vi "AcqDataQSM.vi"(6 "Temp Notifier":refnum<notifier>, 8 "Pressure Notifier":refnum<notifier>, 9 "Lower Notifier":refnum<notifier>, 10 "Upper Notifier":refnum<notifier>, 11 "Acquisition Control":refnum<queue>) -> ()   [LabVIEW 2013, in "main.lvlib"]
doc: "Læser 4 analoge differentierede datakanaler fra ADC'en og skriver dem til en TDMS-fil. Viser 2 af kanaler i grafer og 2 i søjler."
uses:
  main.lvlib
  Controls/Enum Globals.ctl
  Controls/Enum Variables.ctl
  Controls/Enum User Events.ctl
  <vilib>/DAQmx/read.llb/DAQmx Read (Analog 1D DBL NChan 1Samp).vi
  Globals/DataAcqRecordPathGlobal.vi
  <vilib>/DAQmx/miscellaneous.llb/DAQmx Fill In Error Info.vi
panel:
  in  "input cluster":T1
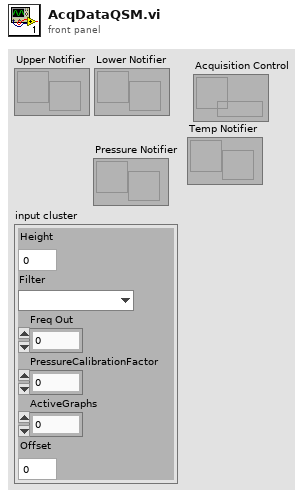
[diagram p1: front panel]
types:
  T1 = cluster{"Height":dbl, "Filter":u16, "Freq Out":i32, "PressureCalibrationFactor":dbl, "ActiveGraphs":u16, "Offset":dbl}
  T2 = typedef "main.lvlib/Enum Globals.ctl" = enum16{"Init", "Set DataPath", "Set Freq", "Get"}
  T3 = typedef "main.lvlib/Enum Variables.ctl" = enum16{"SetAcqFilter", "GetAcqFilter", "Set Filter", "Get Filter", "Set Height", "Get Height", "Set Recorded Height", "Get Recorded Height", "Set Blue Pressure", "Get Blue Pressure", "Set Red Pressure", "Get Red Pressure", "Init", "Reset Pressure", "Set Red Cursors", "Get Red Cursors", "Set Blue Cursors", "Get Blue Cursors", "Set Language", "Get Language", "Set Active Graphs", "Get ActiveGraphs", "Set Method", "Get Method", "Set Encryption", "Get Encryption", "Set ExcelVersion", "Get ExcelVersion", "Set DICOM Avail", "Get DICOM Avail", "Set DICOM Encode", "Get DICOM Encode", "Set JournalExport", "Get JournalExport", "Set Sequence", "Get Sequence", "Set DAQ Connected", "Get DAQ Connected", "Set Current Graph", "Get Current Graph", "Set General Settings", "Get Hyphenation", "Set Arm Calc Method", "Get Arm Calc Method", "Set Dicom Tags", "Get Dicom Tags", "Set BT Serial", "Get BT Serial", "Set BT Accepted Serials", "Get BT Accepted Serials", "Get BT License", "Set BT License"}
  T4 = enum16{"open", "open or create", "create or replace", "create", "open (read-only)"}
  T5 = typedef "main.lvlib/Enum User Events.ctl" = enum16{"User Event", "Init"}
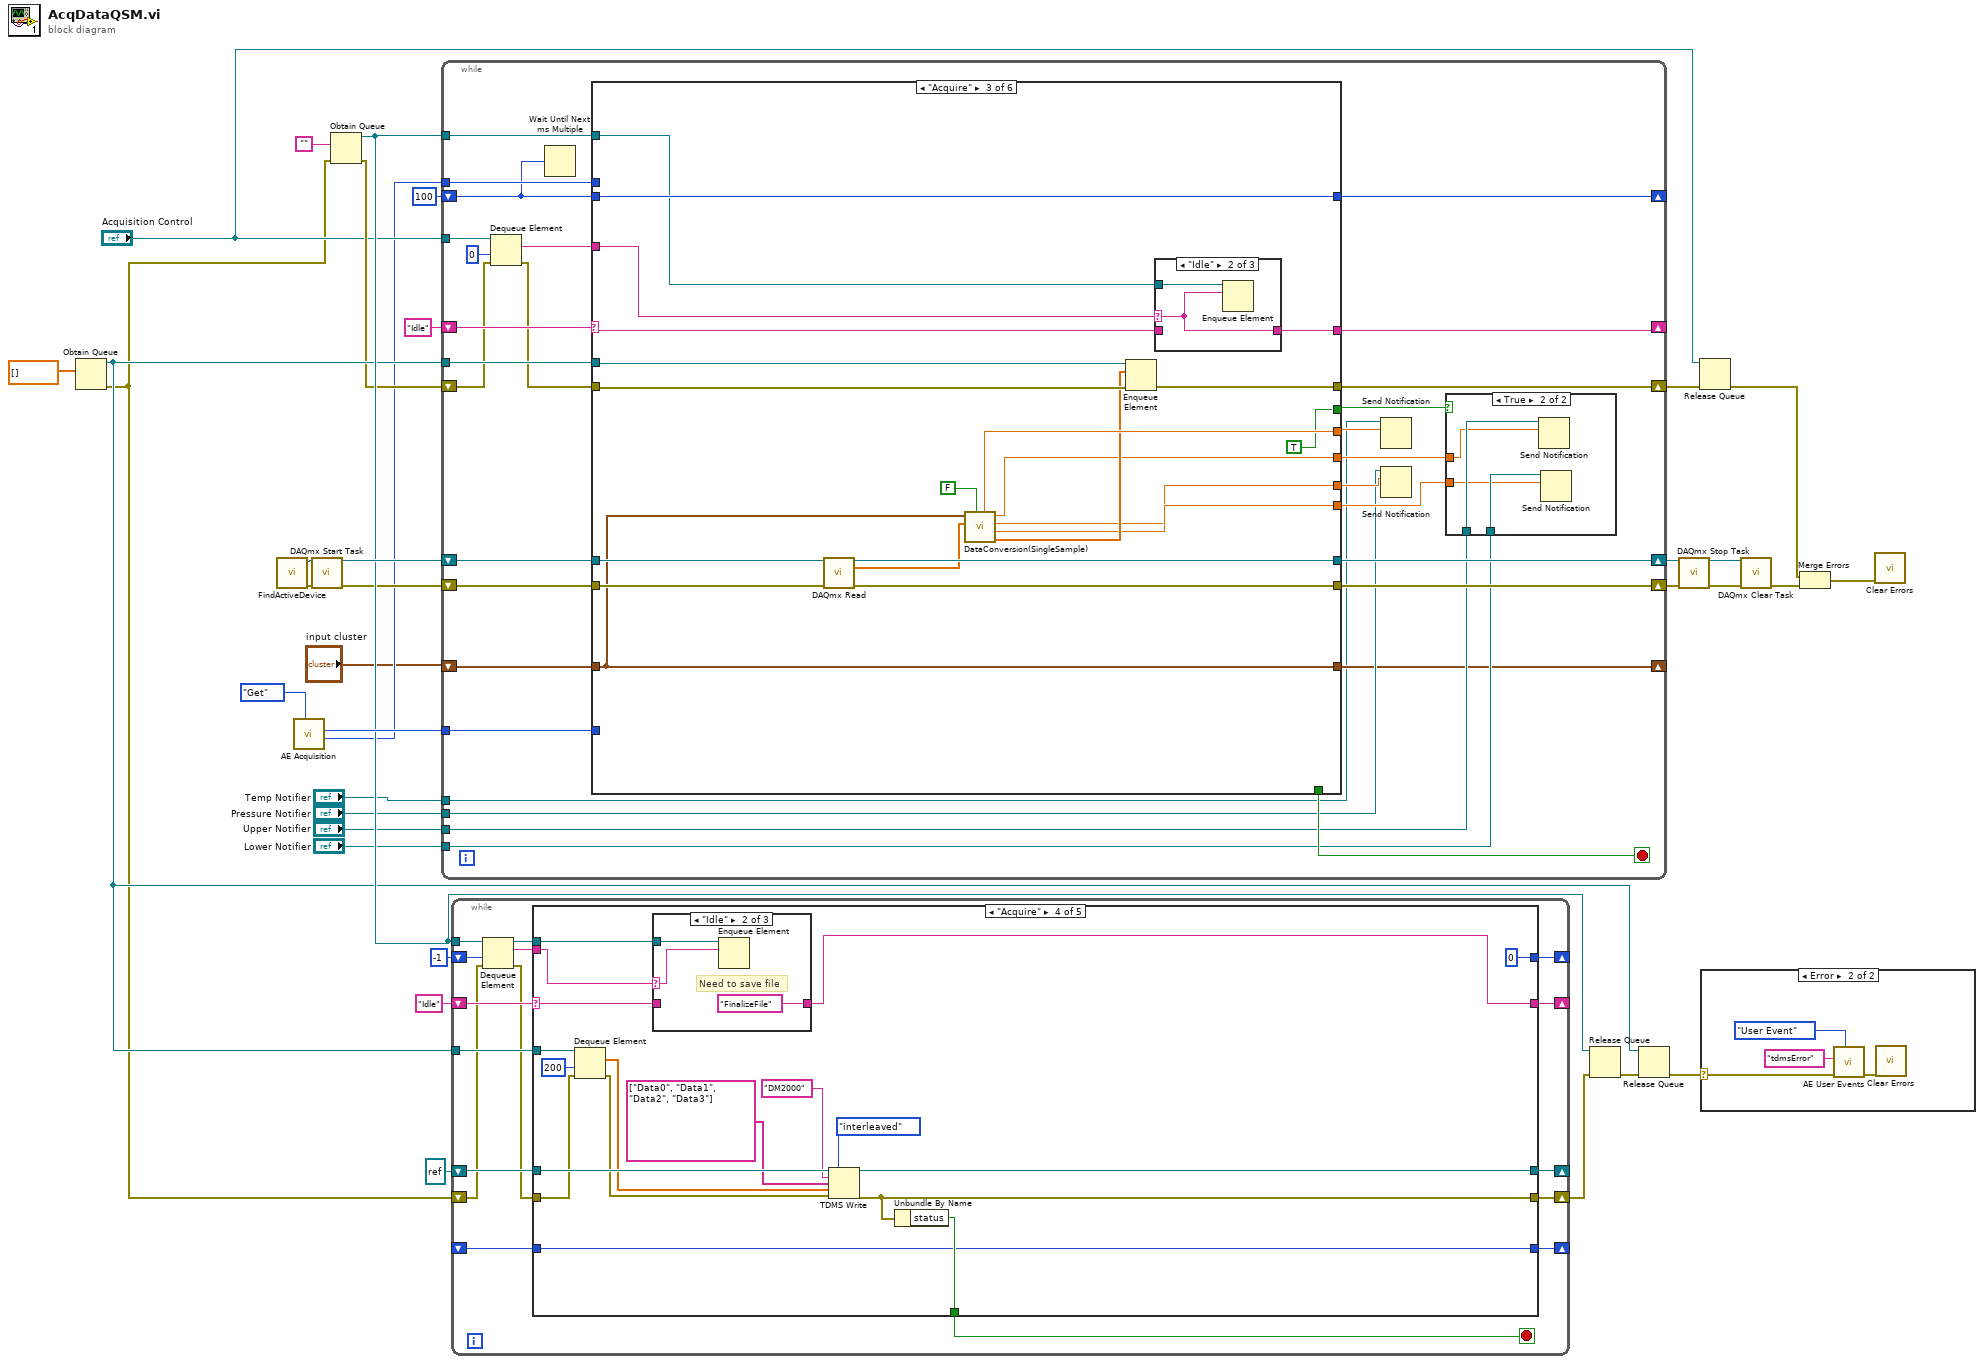
[diagram p0: block diagram]
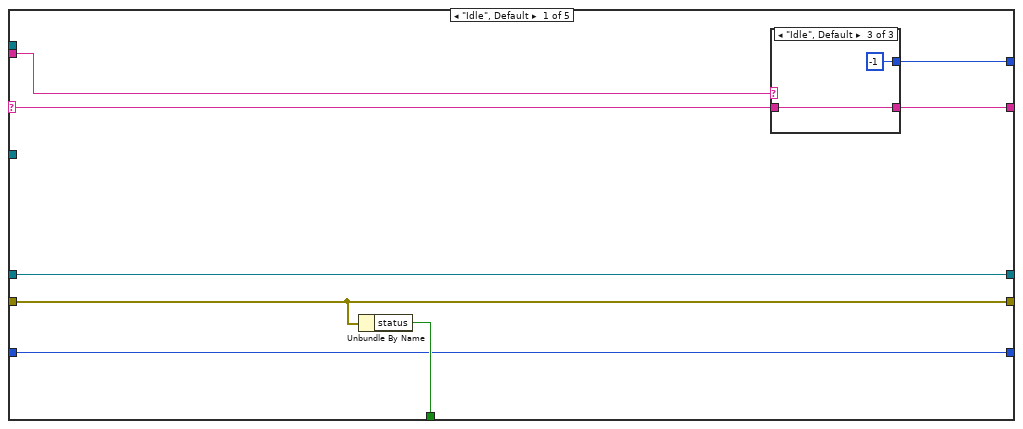
[diagram p3: hidden frame]
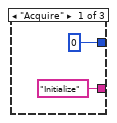
[diagram p4: hidden frame]
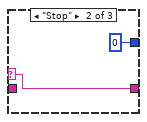
[diagram p5: hidden frame]
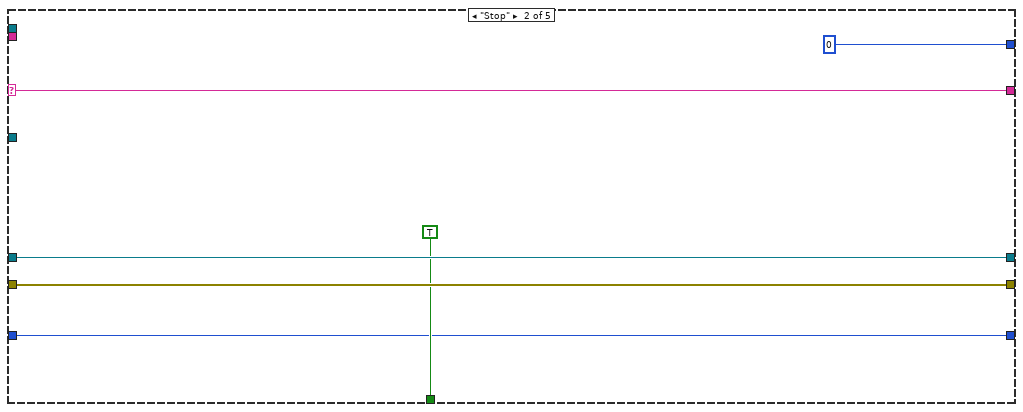
[diagram p6: hidden frame]
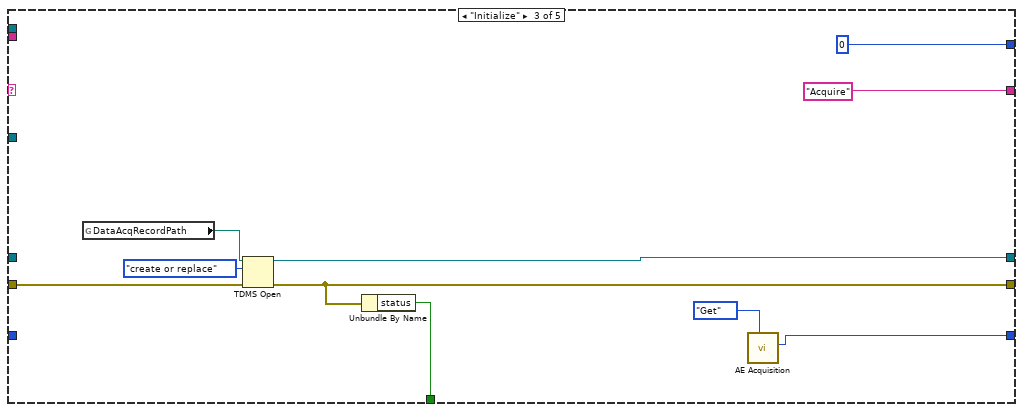
[diagram p7: hidden frame]
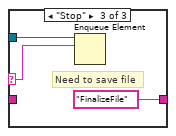
[diagram p9: hidden frame]
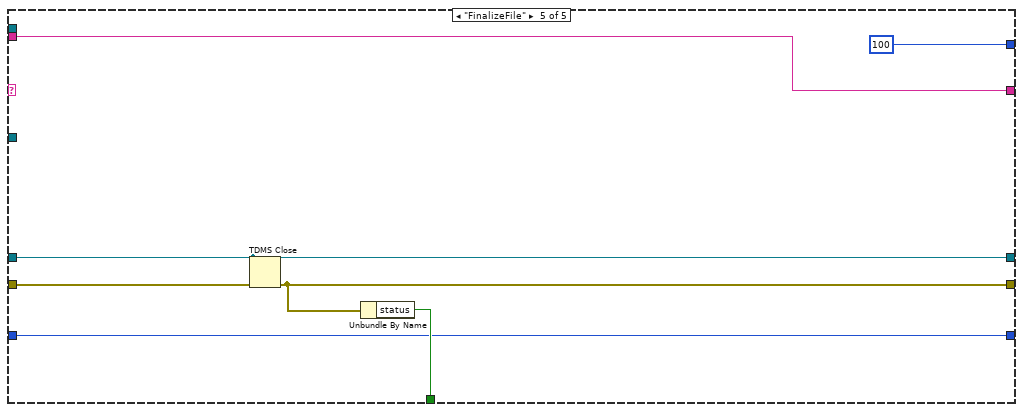
[diagram p10: hidden frame]
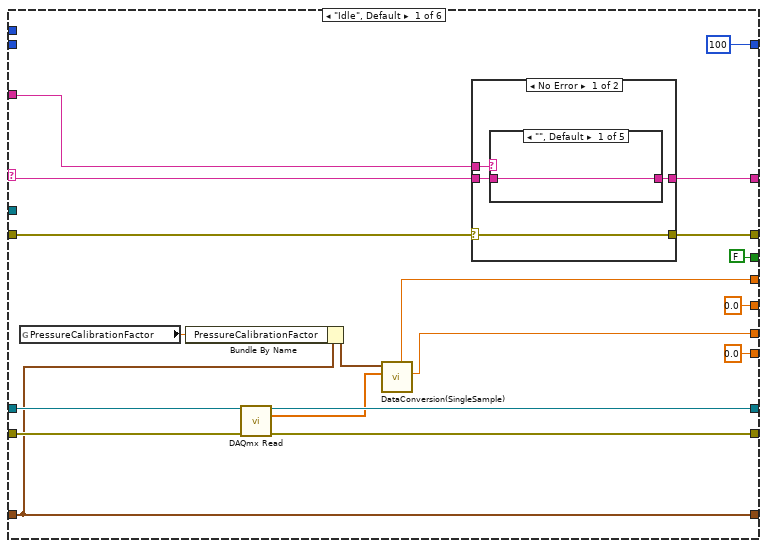
[diagram p12: hidden frame]
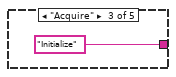
[diagram p14: hidden frame]
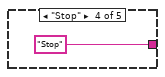
[diagram p15: hidden frame]
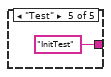
[diagram p16: hidden frame]
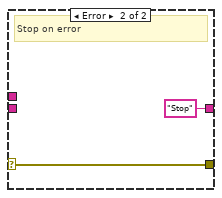
[diagram p17: hidden frame]
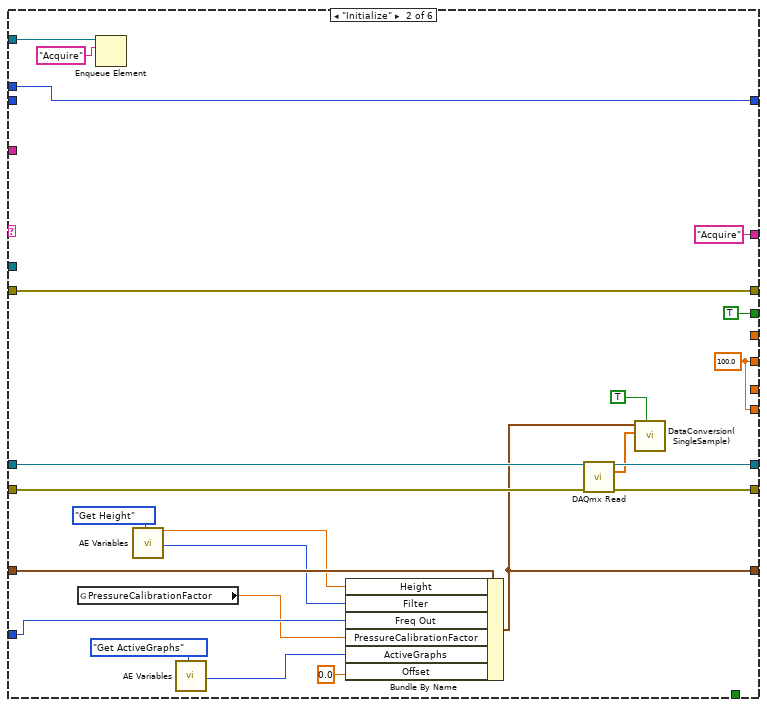
[diagram p18: hidden frame]
diagram:
  n1 = Obtain Queue(element data type=dbl[] []) -> (queue out=w19:refnum<queue>, error out=w7:errorcluster)  [unwired: 4 in, 1 out]
  n2 = call "FindActiveDevice.vi"() -> ("error out"=w22:errorcluster, "task out"=w23:refnum<k21>)  [unwired: 10 in]
  n3 = call "AE Acquisition.vi"("Action"=Enum_Globals."Get") -> ("Period(ms)"=w3:i32, "Freq Out"=w25:i32)  [unwired: 7 in, 2 out]
  n4 = call <vilib>:"DAQmx Start Task.vi"("task/channels in"=w23, "error in"=w22) -> ("task out"=w31:refnum<k21>, "error out"=w16:errorcluster)  [unwired: 12 in]
  n5 = Obtain Queue(element data type="", error in (no error)=w7) -> (queue out=w20:refnum<queue>, error out=w17:errorcluster)  [unwired: 3 in, 1 out]
  n6 = while {
    shift-right: [w46] -> w32
    shift-left: w31 -> [w65]
    shift-right: [w45] -> w35
    shift-left: w16 -> [w64]
    shift-right: [w60] -> _
    shift-left: 100 ("Period(ms)") -> [w44]
    shift-right: [w48] -> w15
    shift-left: w17 -> [w50]
    shift-right: [w61] -> _
    shift-left: "Idle" -> [w62]
    tunnel: w25 -> [w59]
    tunnel: w3 -> [w58]
    shift-right: [w38] -> _
    shift-left: "input cluster" -> [w57]
    tunnel: "Acquisition Control" -> [w53]
    tunnel: w20 -> [w51]
    tunnel: w19 -> [w63]
    tunnel: "Upper Notifier" -> [w42]
    tunnel: "Lower Notifier" -> [w41]
    tunnel: "Pressure Notifier" -> [w39]
    tunnel: "Temp Notifier" -> [w36]
    stop <- w47 stop-if-true
    n7 = Dequeue Element(queue=w53, timeout in ms (-1)=0, error in (no error)=w50) -> (element=w52:string, error out=w49:errorcluster)  [unwired: 2 out]
    n8 = Wait Until Next ms Multiple(millisecond multiple=w44) -> ()  [unwired: 1 out]
    n9 = case shown="\"Acquire\"" w62 {
      selector: w62 -> [w82 _ w135 _ w177 w196]
      tunnel: [w88 w117 w143 w155 w183 w194] -> w45
      tunnel: w65 -> [w87 w118 w142 w156 w182 w195]
      tunnel: [w86 w119 w141 w157 w181 w195] -> w46
      tunnel: w64 -> [w85 w120 w140 w158 w180 w194]
      tunnel: [_ _ _ _ _ TRUE ("status")] -> w47
      tunnel: [100 w114 w134 w152 w171 w193] -> w60
      tunnel: w44 -> [_ _ w134 _ w171 w193]
      tunnel: w63 -> [_ _ w138 _ _ _]
      tunnel: [w70 w111 w125 w167 w176 w188] -> w48
      tunnel: w49 -> [w71 w111 w139 w167 w176 w188]
      tunnel: [w76 _ w130 0.0 w173 _] -> w40
      tunnel: [w84 _ w137 0.0 ("Temperature") w179 _] -> w37
      tunnel: [w81 "Acquire" w136 "Test" w178 w196] -> w61
      tunnel: [0.0 ("Blue Data") w100 w132 _ w174 _] -> w54
      tunnel: [0.0 ("Red Data") w100 w131 _ w175 _] -> w55
      tunnel: [FALSE TRUE TRUE FALSE TRUE FALSE] -> w56
      tunnel: w59 -> [_ w106 _ _ _ _]
      tunnel: w58 -> [_ w114 _ w152 _ _]
      tunnel: w57 -> [w74 w109 w123 w151 w168 w187]
      tunnel: w52 -> [w77 _ w127 _ w170 _]
      tunnel: w51 -> [_ w113 w126 _ _ w190]
      tunnel: [w74 w101 w123 w148 w168 w187] -> w38
      frame "Idle", Default {
        n10 = global read "DataAcqRecordPathGlobal.vi" "PressureCalibrationFactor"() -> (w72:dbl)
        n11 = Bundle By Name(cluster=w74, "PressureCalibrationFactor"=w72) -> (w73:T1)
        n12 = call-poly <vilib>:"DAQmx Read.vi"("task/channels in"=w87, "error in"=w85) -> ("task out"=w86:refnum<k21>, "data"=w75:dbl[], "error out"=w88:errorcluster)  [unwired: 11 in]
        n13 = call "DataConversion(SingleSample).vi"("data"=w75, "input cluster"=w73) -> ("Temperature"=w84:dbl, "Pressure"=w76:dbl)  [unwired: 4 in, 3 out]
        n14 = case shown="No Error" w71 {
          selector: w71 -> [w89 w98]
          tunnel: w82 -> [w92 _]
          tunnel: [w91 "Stop"] -> w81
          tunnel: w77 -> [w90 _]
          tunnel: [w89 w98] -> w70
          frame No Error {
            n15 = case shown="\"\", Default" w90 {
              tunnel: w92 -> [w93 w94 _ _ _]
              tunnel: [w93 w94 "Initialize" "Stop" "InitTest"] -> w91
              frame "", Default {
              }
              frame "Idle" {
              }
              frame "Acquire" {
              }
              frame "Stop" {
              }
              frame "Test" {
              }
            }
          }
          frame Error {
            # "Stop on error"
          }
        }
      }
      frame "Initialize" {
        w100 = 100.0 ("Blue Data")
        n16 = global read "DataAcqRecordPathGlobal.vi" "PressureCalibrationFactor"() -> (w105:dbl)
        n17 = Enqueue Element(queue=w113, element="Acquire") -> ()  [unwired: 2 in, 3 out]
        n18 = call "AE Variables.vi"("Action"=Enum_Variables."Get Height") -> ("NumericOut"=w102:dbl, "RingOut"=w103:u16)  [unwired: 11 in, 6 out]
        n19 = call "AE Variables.vi"("Action"=Enum_Variables."Get ActiveGraphs") -> ("RingOut"=w104:u16)  [unwired: 11 in, 7 out]
        n20 = Bundle By Name(cluster=w109, "Height"=w102, "Filter"=w103, "Freq Out"=w106, "PressureCalibrationFactor"=w105, "ActiveGraphs"=w104, "Offset"=0.0) -> (w101:T1)
        n21 = call-poly <vilib>:"DAQmx Read.vi"("task/channels in"=w118, "error in"=w120) -> ("task out"=w119:refnum<k21>, "data"=w108:dbl[], "error out"=w117:errorcluster)  [unwired: 11 in]
        n22 = call "DataConversion(SingleSample).vi"("data"=w108, "input cluster"=w101, "Init"=TRUE) -> ()  [unwired: 3 in, 5 out]
      }
      frame "Acquire" {
        n23 = call-poly <vilib>:"DAQmx Read.vi"("task/channels in"=w142, "error in"=w140) -> ("task out"=w141:refnum<k21>, "data"=w124:dbl[], "error out"=w143:errorcluster)  [unwired: 11 in]
        n24 = call "DataConversion(SingleSample).vi"("data"=w124, "input cluster"=w123, "Init"=FALSE) -> ("Temperature"=w137:dbl, "All Data"=w133:dbl[], "Red Data"=w131:dbl, "Pressure"=w130:dbl, "Blue Data"=w132:dbl)  [unwired: 3 in]
        n25 = Enqueue Element(queue=w138, element=w133, error in (no error)=w139) -> (error out=w125:errorcluster)  [unwired: 1 in, 2 out]
        n26 = case shown="\"Idle\"" w127 {
          selector: w127 -> [_ w145 w147]
          tunnel: [w144 w145 w147] -> w136
          tunnel: w135 -> [w144 _ _]
          tunnel: w126 -> [_ w146 _]
          frame "", Default {
          }
          frame "Idle" {
            n27 = Enqueue Element(queue=w146, element=w145) -> ()  [unwired: 2 in, 3 out]
          }
          frame "Stop" {
          }
        }
      }
      frame "InitTest" {
        n28 = call "AE Variables.vi"("Action"=Enum_Variables."Get ActiveGraphs") -> ("RingOut"=w149:u16)  [unwired: 11 in, 7 out]
        n29 = Bundle By Name(cluster=w151, "ActiveGraphs"=w149) -> (w148:T1)
        n30 = call-poly <vilib>:"DAQmx Read.vi"("task/channels in"=w156, "error in"=w158) -> ("task out"=w157:refnum<k21>, "data"=w150:dbl[], "error out"=w155:errorcluster)  [unwired: 11 in]
        n31 = call "DataConversion(SingleSample).vi"("data"=w150, "input cluster"=w148, "Init"=TRUE) -> ("Red Data"=w160:dbl, "Blue Data"=w161:dbl)  [unwired: 3 in, 3 out]
        n32 = Build Array(w161, w160) -> (w159:dbl[])
        n33 = call "AdjustScalesInterval.vi"("Action"=enum16{"Init", "Set Scale"}."Init", "Data"=w159) -> ()  [unwired: 10 in]
      }
      frame "Test" {
        n34 = call-poly <vilib>:"DAQmx Read.vi"("task/channels in"=w182, "error in"=w180) -> ("task out"=w181:refnum<k21>, "data"=w169:dbl[], "error out"=w183:errorcluster)  [unwired: 11 in]
        n35 = call "DataConversion(SingleSample).vi"("data"=w169, "input cluster"=w168) -> ("Temperature"=w179:dbl, "Red Data"=w175:dbl, "Pressure"=w173:dbl, "Blue Data"=w174:dbl)  [unwired: 4 in, 1 out]
        n36 = case shown="\"False\", Default" w170 {
          tunnel: [w184 "Idle" "Stop"] -> w178
          tunnel: w177 -> [w184 _ _]
          frame "False", Default {
          }
          frame "Idle" {
          }
          frame "Stop" {
          }
        }
      }
      frame "Stop" {
        n37 = Enqueue Element(queue=w190, element="Stop") -> ()  [unwired: 2 in, 3 out]
      }
    }
    n38 = Send Notification(notification=w37, notifier=w36) -> ()  [unwired: 1 in, 2 out]
    n39 = Send Notification(notification=w40, notifier=w39) -> ()  [unwired: 1 in, 2 out]
    n40 = case shown="True" w56 {
      tunnel: w55 -> [_ w67]
      tunnel: w54 -> [_ w66]
      tunnel: w42 -> [_ w69]
      tunnel: w41 -> [_ w68]
      frame False {
      }
      frame True {
        n41 = Send Notification(notification=w66, notifier=w69) -> ()  [unwired: 1 in, 2 out]
        n42 = Send Notification(notification=w67, notifier=w68) -> ()  [unwired: 1 in, 2 out]
      }
    }
  }
  n43 = while {
    tunnel: w19 -> [w212]
    shift-right: [w210] -> _
    shift-left: refnum<k34> refnum ("tdms file out") -> [w211]
    shift-right: [w209] -> w27
    shift-left: w7 -> [w199]
    shift-right: [w206] -> _
    shift-left: "Idle" -> [w207]
    shift-right: [w205] -> _
    shift-left: _ -> [w204]
    tunnel: w20 -> [w203]
    shift-right: [w200] -> _
    shift-left: -1 -> [w201]
    stop <- w208 stop-if-true
    n44 = Dequeue Element(queue=w203, timeout in ms (-1)=w201, error in (no error)=w199) -> (queue out=w197:refnum<queue>, element=w202:string, error out=w198:errorcluster)  [unwired: 1 out]
    n45 = case shown="\"Acquire\"" w207 {
      selector: w207 -> [w218 w232 _ w255 _]
      tunnel: w212 -> [_ _ _ w256 _]
      tunnel: w211 -> [w220 w231 _ w259 w271]
      tunnel: [w220 w231 w237 w260 w271] -> w210
      tunnel: [w217 w230 w238 w258 w272] -> w209
      tunnel: w198 -> [w217 w230 w240 w252 w274]
      tunnel: [w216 TRUE ("status") w239 w257 w273] -> w208
      tunnel: [w219 w232 "Acquire" w249 w268] -> w206
      tunnel: [w215 w228 w234 w247 w270] -> w205
      tunnel: w204 -> [w215 w228 _ w247 w270]
      tunnel: w202 -> [w214 _ _ w245 w268]
      tunnel: [w213 0 0 0 100] -> w200
      tunnel: w197 -> [_ _ _ w244 _]
      frame "Idle", Default {
        n46 = Unbundle By Name(w217) -> ("status"=w216:bool)
        n47 = case shown="\"Idle\", Default" w214 {
          selector: w214 -> [_ w223 _]
          tunnel: ["Initialize" w223 w226] -> w219
          tunnel: w218 -> [_ _ w226]
          tunnel: [0 0 -1] -> w213
          frame "Acquire" {
          }
          frame "Stop" {
          }
          frame "Idle", Default {
          }
        }
      }
      frame "Stop" {
      }
      frame "Initialize" {
        n48 = global read "DataAcqRecordPathGlobal.vi" "DataAcqRecordPath"() -> (w242:path)
        n49 = TDMS Open(8:w240, 10:T4."create or replace" ("operation (0:open)"), 11:w242) -> (0:w238:errorcluster, 3:w237:refnum<k34>)  [unwired: 4 in]
        n50 = Unbundle By Name(w238) -> ("status"=w239:bool)
        n51 = call "AE Acquisition.vi"("Action"=Enum_Globals."Get") -> ("Freq Out"=w234:i32)  [unwired: 7 in, 3 out]
      }
      frame "Acquire" {
        n52 = Dequeue Element(queue=w256, timeout in ms (-1)=200, error in (no error)=w252) -> (element=w248:dbl[], error out=w251:errorcluster)  [unwired: 2 out]
        n53 = case shown="\"Idle\"" w245 {
          selector: w245 -> [_ w262 w265]
          tunnel: [w261 "FinalizeFile" "FinalizeFile"] -> w249
          tunnel: w255 -> [w261 _ _]
          tunnel: w244 -> [_ w263 w266]
          frame "", Default {
          }
          frame "Idle" {
            # "Need to save file"
            n54 = Enqueue Element(queue=w263, element=w262) -> ()  [unwired: 2 in, 3 out]
          }
          frame "Stop" {
            # "Need to save file"
            n55 = Enqueue Element(queue=w266, element=w265) -> ()  [unwired: 2 in, 3 out]
          }
        }
        n56 = TDMS Write(0:w259, 1:enum16{"decimated", "interleaved"}."interleaved" ("data layout (0:decimated)"), 5:"DM2000", 7:string[] ["Data0", "Data1", "Data2", "Data3"], 9:w248, 11:w251) -> (4:w260:refnum<k34>, 15:w258:errorcluster)  [unwired: 2 out]
        n57 = Unbundle By Name(w258) -> ("status"=w257:bool)
      }
      frame "FinalizeFile" {
        n58 = TDMS Close(8:w274, 11:w271) -> (0:w272:errorcluster)  [unwired: 1 out]
        n59 = Unbundle By Name(w272) -> ("status"=w273:bool)
      }
    }
  }
  n60 = Release Queue(queue=w20, error in (no error)=w27) -> (error out=w18:errorcluster)  [unwired: 1 in, 2 out]
  n61 = Release Queue(queue=w19, error in (no error)=w18) -> (error out=w13:errorcluster)  [unwired: 1 in, 2 out]
  n62 = call <vilib>:"DAQmx Stop Task.vi"("task/channels in"=w32, "error in"=w35) -> ("task out"=w34:refnum<k21>, "error out"=w33:errorcluster)  [unwired: 12 in]
  n63 = Release Queue(queue="Acquisition Control", error in (no error)=w15) -> (error out=w11:errorcluster)  [unwired: 1 in, 2 out]
  n64 = case shown="Error" w13 {
    selector: w13 -> [_ w276]
    frame No Error {
    }
    frame Error {
      n65 = call "AE User Events.vi"("Action"=Enum_User_Events."User Event", "error in (no error)"=w276, "User Event"="tdmsError") -> ("error out"=w275:errorcluster)  [unwired: 7 in, 1 out]
      n66 = call <vilib>:"Clear Errors.vi"("error in (no error)"=w275) -> ()  [unwired: 6 in, 1 out]
    }
  }
  n67 = call <vilib>:"DAQmx Clear Task.vi"("task in"=w34, "error in"=w33) -> ("error out"=w12:errorcluster)  [unwired: 13 in]
  n68 = Merge Errors(w11, w12) -> (w10:errorcluster)
  n69 = call <vilib>:"Clear Errors.vi"("error in (no error)"=w10) -> ()  [unwired: 6 in, 1 out]
